vi "GRBL INFO.vi"(8 "error in (no error)":errorcluster, 11 "Cluster in":T1) -> (0 "error out":errorcluster, 1 "GRBL VERSION":string, 2 "Cluster out":T1, 3 "GRBL CURRENT CONFIG":string)   [LabVIEW 2021]
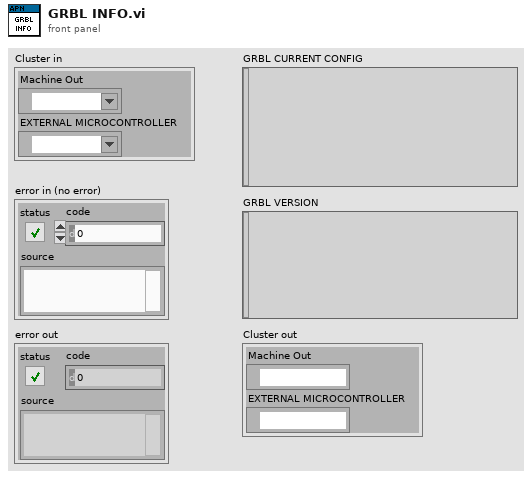
[diagram p1: front panel]
types:
  T1 = cluster{"Machine Out":refnum<visa-resource-name>, "EXTERNAL MICROCONTROLLER":refnum<visa-resource-name>}
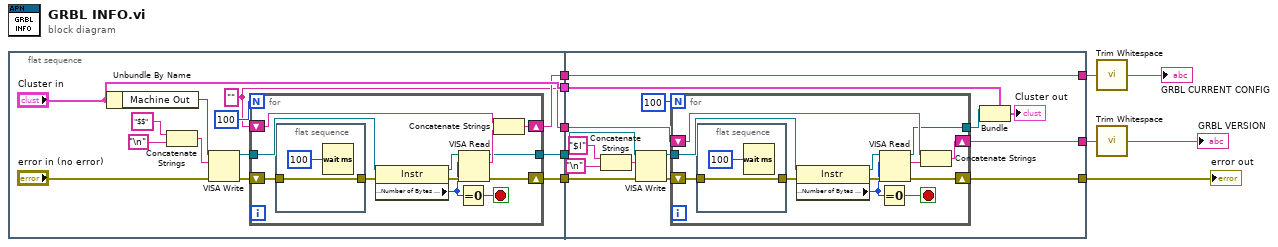
[diagram p0: block diagram]
diagram:
  n1 = flat-sequence {
    tunnel: ["Cluster in"] -> w9
    tunnel: [w22] -> w8
    tunnel: [w11] -> w7
    tunnel: [w16] -> w6
    tunnel: [w13] -> w5
    tunnel: w9 -> [w47]
    tunnel: w8 -> [w44]
    tunnel: w7 -> [w45]
    tunnel: w6 -> [w42]
    tunnel: [w43] -> w4
    tunnel: [w42] -> w2
    tunnel: [w38] -> w10
    tunnel: w5 -> [w40]
    frame #0 {
      w11 = ""
      n2 = Unbundle By Name("Cluster in") -> ("Machine Out"=w17:refnum<visa-resource-name>)
      n3 = Concatenate Strings("$$" ("string"), "\n") -> (w18:string)
      n4 = VISA Write(VISA resource name=w17, write buffer=w18, error in (no error)="error in (no error)") -> (VISA resource name out=w20:refnum<visa-resource-name>, error out=w14:errorcluster)  [unwired: 1 out]
      n5 = for {
        N: 100 -> [_]
        tunnel: w20 -> [w33]
        shift-right: [w35] -> w16
        shift-left: w11 -> [w34]
        tunnel: [w30] -> w22
        shift-right: [w28] -> w13
        shift-left: w14 -> [w26]
        stop <- w27 stop-if-true
        n6 = flat-sequence {
          tunnel: w26 -> [w36]
          tunnel: [w36] -> w25
          frame #0 {
            n7 = Wait (ms)(milliseconds to wait=u32 100) -> ()  [unwired: 1 out]
          }
        }
        n8 = property class="Instr"(reference=w33, error in=w25) -> (reference out=w31:refnum<visa-resource-name>, error out=w29:errorcluster, "Serial Settings:Number of Bytes at Serial Port"=w24:u32)
        n9 = Equal To 0?(x=w24) -> (x = 0?=w27:bool)
        n10 = VISA Read(VISA resource name=w31, byte count=w24, error in (no error)=w29) -> (VISA resource name out=w30:refnum<visa-resource-name>, read buffer=w32:string, error out=w28:errorcluster)  [unwired: 1 out]
        n11 = Concatenate Strings(w34, w32) -> (w35:string)
      }
    }
    frame #1 {
      n12 = Concatenate Strings("$I" ("string"), "\n") -> (w52:string)
      n13 = VISA Write(VISA resource name=w44, write buffer=w52, error in (no error)=w40) -> (VISA resource name out=w51:refnum<visa-resource-name>, error out=w39:errorcluster)  [unwired: 1 out]
      n14 = for {
        N: 100 -> [_]
        tunnel: w51 -> [w62]
        shift-right: [w64] -> w43
        shift-left: w45 -> [w63]
        tunnel: [w59] -> w50
        shift-right: [w57] -> w38
        shift-left: w39 -> [w55]
        stop <- w56 stop-if-true
        n15 = flat-sequence {
          tunnel: w55 -> [w65]
          tunnel: [w65] -> w54
          frame #0 {
            n16 = Wait (ms)(milliseconds to wait=u32 100) -> ()  [unwired: 1 out]
          }
        }
        n17 = property class="Instr"(reference=w62, error in=w54) -> (reference out=w60:refnum<visa-resource-name>, error out=w58:errorcluster, "Serial Settings:Number of Bytes at Serial Port"=w53:u32)
        n18 = Equal To 0?(x=w53) -> (x = 0?=w56:bool)
        n19 = VISA Read(VISA resource name=w60, byte count=w53, error in (no error)=w58) -> (VISA resource name out=w59:refnum<visa-resource-name>, read buffer=w61:string, error out=w57:errorcluster)  [unwired: 1 out]
        n20 = Concatenate Strings(w63, w61) -> (w64:string)
      }
      n21 = Bundle(cluster=w47, "Machine Out"=w50) -> (→"Cluster out":T1)  [unwired: 1 in]
    }
  }
  n22 = call <vilib>:"Trim Whitespace.vi"("string"=w2) -> ("trimmed string"=→"GRBL CURRENT CONFIG":string)  [unwired: 1 in]
  n23 = call <vilib>:"Trim Whitespace.vi"("string"=w4) -> ("trimmed string"=→"GRBL VERSION":string)  [unwired: 1 in]
  "error out" <- w10
